vi "CreateGetSetSerializableVIs.vi"(4 "SaveTo Path":path, 6 "Template VI path":path, 7 "Type":T1, 8 "error in (no error)":errorcluster, 10 "Application":refnum<vi>, 11 "LVClassLibrary Ref":refnum<vi>) -> (0 "error out":errorcluster, 2 "Application":refnum<vi>, 3 "LVClassLibrary Ref":refnum<vi>)   [LabVIEW 2019, in "BlueSerializationScripts.lvlib"]
uses:
  BlueSerializationScripts.lvlib
  AccessDirection.ctl
  BlueUtilityScripts/GetDescendantOptions.ctl
  BlueSerialVirtualFolders.ctl
  5ef38f9a-c5da-4de2-91f0-a49638afd19c.vi
  <userlib>/_OpenG.lib/file/file.llb/File Exists - Scalar__ogtk.vi
  BlueUtilityScripts/BlueUtilityScripts.lvlib
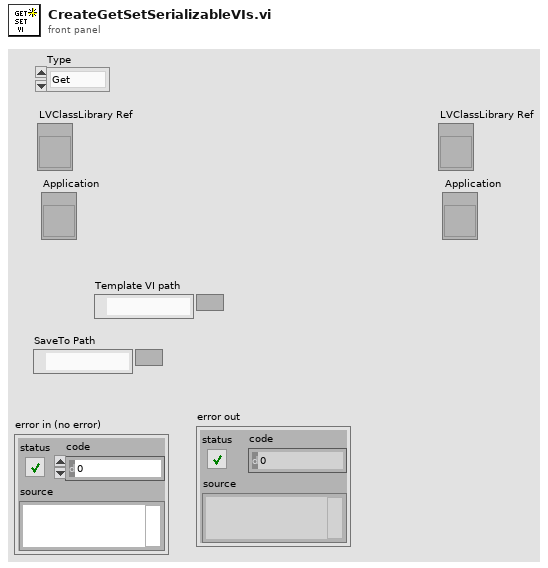
[diagram p1: front panel]
types:
  T1 = typedef "BlueSerializationScripts.lvlib/AccessDirection.ctl" = enum16{"Get", "Set"}
  T2 = typedef "BlueSerializationScripts.lvlib/BlueSerialVirtualFolders.ctl" = enum16{"BlueSerialization", "Mutations"}
  T3 = typedef "BlueUtilityScripts.lvlib/GetDescendantOptions.ctl" = cluster{"Type":string, "ExcludeDependencies":bool, "ExcludeBuilds":bool, "ExcludeTargets":bool}
  T4 = enum32{"invalid scope", "public", "private", "protected", "community"}
  T5 = enum32{"invalid VI type", "Standard VI", "Control VI", "Global VI", "Polymorphic VI", "Configuration VI", "SubSystem", "Facade VI", "Method VI"}
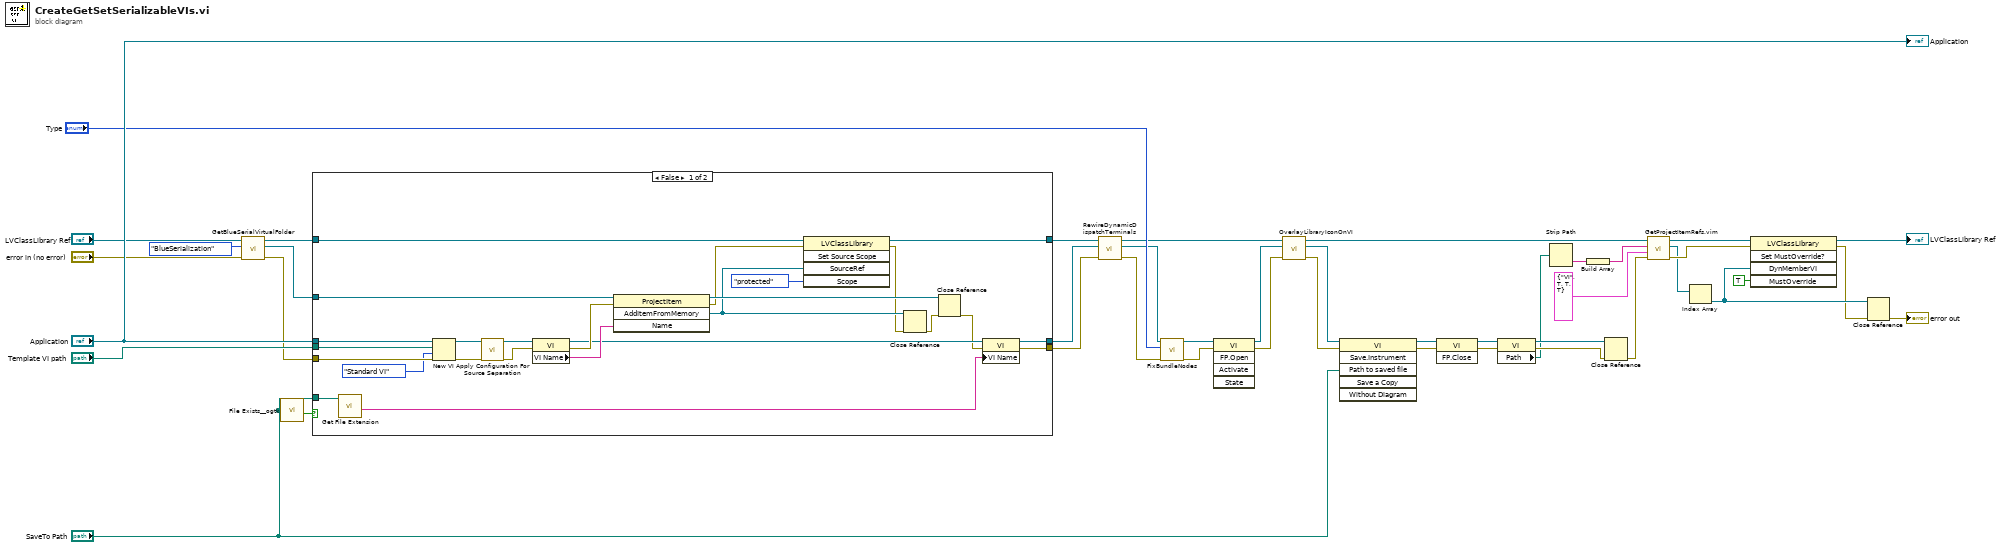
[diagram p0: block diagram]
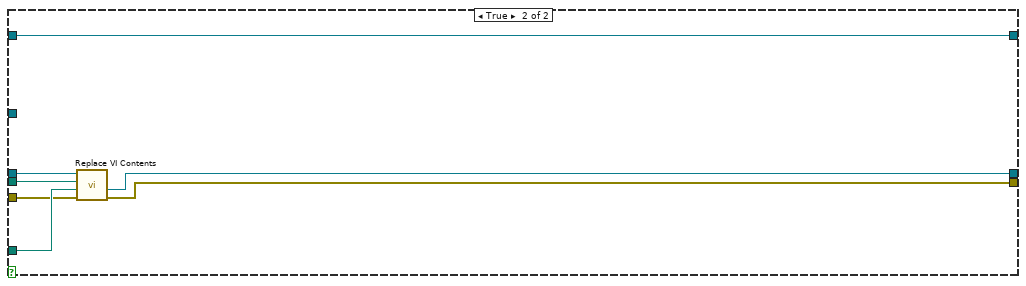
[diagram p2: hidden frame]
diagram:
  n1 = call "GetBlueSerialVirtualFolder.vi"("error in (no error)"="error in (no error)", "Virtual Folder"=BlueSerialVirtualFolders."BlueSerialization", "LVClassLibrary Ref"="LVClassLibrary Ref") -> ("error out"=w15:errorcluster, "Folder Refnum out"=w14:refnum<vi>, "LVClassLibrary Ref"=w2:refnum<vi>)  [unwired: 6 in]
  n2 = call-poly <userlib>:"File Exists__ogtk.vi"("file path"="SaveTo Path") -> ("exists"=w35:bool)  [unwired: 6 in, 1 out]
  n3 = case shown="False" w35 {
    tunnel: "Application" -> [w68 w75]
    tunnel: "Template VI path" -> [w67 w74]
    tunnel: [w62 w71] -> w12
    tunnel: w14 -> [w61 _]
    tunnel: w15 -> [w59 w72]
    tunnel: [w57 w70] -> w11
    tunnel: "SaveTo Path" -> [w51 w73]
    tunnel: w2 -> [w48 w69]
    tunnel: [w44 w69] -> w1
    frame False {
      n4 = call <vilib>:"Get File Extension.vi"("file"=w51) -> ("filename without extension"=w60:string)  [unwired: 6 in, 4 out]
      n5 = New VI(8:w59, 9:T5."Standard VI" ("vi type (standard vi)"), 10:w67, 11:w68) -> (0:w53:errorcluster, 3:w54:refnum<vi>)  [unwired: 3 out]
      n6 = call <vilib>:"Apply Configuration For Source Separation.vi"("error in (no error)"=w53, "VI in"=w54) -> ("error out"=w58:errorcluster, "VI out"=w63:refnum<vi>)  [unwired: 8 in]
      n7 = property class="VI"(reference=w63, error in=w58) -> (reference out=w64:refnum<vi>, error out=w66:errorcluster, "VI Name"=w65:string)
      n8 = invoke class="ProjectItem" method="AddItemFromMemory"(reference=w61, error in=w66, "Name"=w65) -> (reference out=w55:refnum<vi>, error out=w47:errorcluster, "AddItemFromMemory"=w46:refnum<vi>)  [unwired: 1 in, 1 out]
      n9 = invoke class="LVClassLibrary" method="Set Source Scope"(reference=w48, error in=w47, "SourceRef"=w46, "Scope"=T4."protected" ("scope")) -> (reference out=w44:refnum<vi>, error out=w45:errorcluster)  [unwired: 1 in, 3 out]
      n10 = Close Reference(reference=w46, error in (no error)=w45) -> (error out=w50:errorcluster)
      n11 = Close Reference(reference=w55, error in (no error)=w50) -> (error out=w56:errorcluster)
      n12 = property class="VI"(reference=w64, error in=w56, "VI Name"=w60) -> (reference out=w62:refnum<vi>, error out=w57:errorcluster)
    }
    frame True {
      n13 = call "Replace VI Contents.vi"("error in (no error)"=w72, "Target VI"=w73, "Template VI"=w74, "Application"=w75) -> ("error out"=w70:errorcluster, "Target vi refnum"=w71:refnum<vi>)  [unwired: 5 in, 1 out]
    }
  }
  n14 = call "RewireDynamicDispatchTerminals.vi"("error in (no error)"=w11, "VI Reference"=w12, "LVClassLibrary"=w1) -> ("error out"=w10:errorcluster, "VI Reference"=w9:refnum<vi>, "LVClassLibrary"=w8:refnum<vi>)  [unwired: 6 in]
  n15 = call "FixBundleNodes.vi"("error in (no error)"=w10, "Type"="Type", "VI Refnum"=w9) -> ("error out"=w39:errorcluster, "VI Refnum"=w40:refnum<vi>)  [unwired: 7 in]
  n16 = invoke class="VI" method="FP.Open"(reference=w40, error in=w39) -> (reference out=w6:refnum<vi>, error out=w5:errorcluster)  [unwired: 3 in, 3 out]
  n17 = call "OverlayLibraryIconOnVI.vi"("error in (no error)"=w5, "VI Refnum out"=w6, "LVClassLibrary"=w8) -> ("error out"=w4:errorcluster, "VI Refnum out"=w3:refnum<vi>, "LVClassLibrary"=w7:refnum<vi>)  [unwired: 5 in, 1 out]
  n18 = invoke class="VI" method="Save.Instrument"(reference=w3, error in=w4, "Path to saved file"="SaveTo Path") -> (reference out=w38:refnum<vi>, error out=w37:errorcluster)  [unwired: 3 in, 4 out]
  n19 = invoke class="VI" method="FP.Close"(reference=w38, error in=w37) -> (reference out=w34:refnum<vi>, error out=w33:errorcluster)  [unwired: 1 in, 1 out]
  n20 = property class="VI"(reference=w34, error in=w33) -> (reference out=w32:refnum<vi>, error out=w31:errorcluster, "Path"=w20:path)
  n21 = Strip Path(path=w20) -> (name=w19:string)  [unwired: 1 out]
  n22 = Build Array(w19) -> (w30:string[])
  n23 = Close Reference(reference=w32, error in (no error)=w31) -> (error out=w25:errorcluster)
  n24 = call "GetProjectItemRefs.vim"("error in (no error)"=w25, "Search Options"=T3 {"Type"="VI", "ExcludeDependencies"=TRUE, "ExcludeBuilds"=TRUE, "ExcludeTargets"=TRUE}, "Item Name"=w30, "ProjectItem"=w7) -> ("error out"=w28:errorcluster, "Item Refs"=w27:refnum<vi>[], "ProjectItem"=w18:refnum<vi>)  [unwired: 4 in, 1 out]
  n25 = Index Array(array=w27) -> (element=w24:refnum<vi>)  [unwired: 1 in]
  n26 = invoke class="LVClassLibrary" method="Set MustOverride?"(reference=w18, error in=w28, "DynMemberVI"=w24, "MustOverride"=TRUE ("Must Override?")) -> (reference out=→"LVClassLibrary Ref":refnum<vi>, error out=w23:errorcluster)  [unwired: 1 in, 3 out]
  n27 = Close Reference(reference=w24, error in (no error)=w23) -> (error out=→"error out":errorcluster)
  "Application" <- "Application"
